vi "BeautifyCardImage.vi"(11 "Image URL":string="http://forums.ni.com/legacyfs/online/20297_Labview-logo1.jpg") -> (3 "Resized image":picture)   [LabVIEW 2020, in "StashRoyale.lvclass"]
uses:
  StashRoyale.lvclass
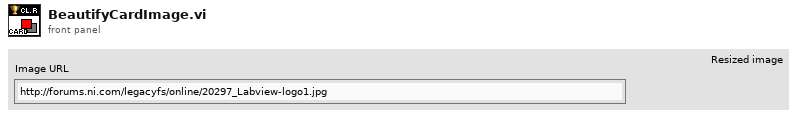
[diagram p1: front panel]
types:
  T1 = typedef "LVBoundsTypeDef.ctl" = cluster{"Width":u32, "Height":u32}
  T2 = typedef "imagedata.ctl" = cluster{"image type":i32, "image depth":i32, "image":u8[], "mask":u8[], "colors":u32[], "Rectangle":cluster{"left":i16, "top":i16, "right":i16, "bottom":i16}}
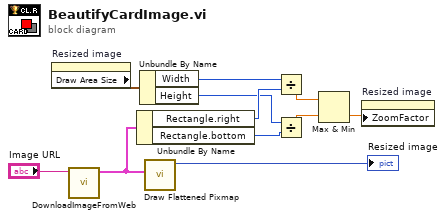
[diagram p0: block diagram]
diagram:
  n1 = property on="Resized image" class="Pict"() -> ("Draw Area Size"=w11:T1)  [unwired: 2 in, 2 out]
  n2 = call "DownloadImageFromWeb.vi"("Image URL"="Image URL") -> ("Downloaded Image"=w10:T2)  [unwired: 9 in, 1 out]
  n3 = Unbundle By Name(w10) -> ("Rectangle.right"=w8:i16, "Rectangle.bottom"=w7:i16)
  n4 = Unbundle By Name(w11) -> ("Width"=w9:u32, "Height"=w6:u32)
  n5 = call <vilib>:"Draw Flattened Pixmap.vi"("image data"=w10) -> ("new picture"=→"Resized image":picture)  [unwired: 8 in]
  n6 = Divide(x=w9, y=w8) -> (x/y=w4:dbl)
  n7 = Divide(x=w6, y=w7) -> (x/y=w5:dbl)
  n8 = Max & Min(x=w4, y=w5) -> (min(x,y)=w3:dbl)  [unwired: 1 out]
  n9 = property on="Resized image" class="Pict"("ZoomFactor"=w3) -> ()  [unwired: 2 in, 2 out]
